vi "Configure.vi"(8 "error in (no error)":errorcluster, 11 "navX - SERIAL in":refnum<class "navX - SERIAL.lvclass">) -> (0 "error out":errorcluster, 3 "navX - SERIAL out":refnum<class "navX - SERIAL.lvclass">)   [LabVIEW 2015, in "navX Library v3.lvlib" / "navX - SERIAL.lvclass"]
uses:
  navX - SERIAL.lvclass
  ProtocolID.ctl
  _NI WPI Serial USB/WPI_SerialPort_USB.ctl
  navX - SERIAL.lvclass/navX - SERIAL.ctl
  navX - Base/navX - Base.lvclass/navX - Base.ctl
  navX - Base/navX - Base.lvclass
  _NI WPI Serial USB/_NI WPI Serial USB.lvlib
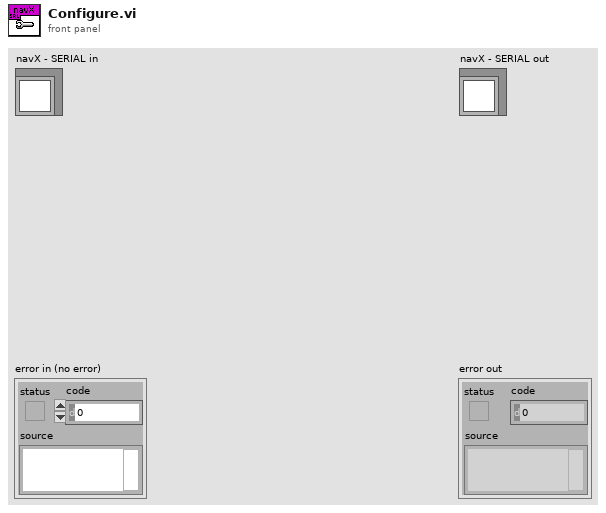
[diagram p1: front panel]
types:
  T1 = typedef "_NI WPI Serial USB.lvlib/WPI_SerialPort_USB.ctl" = enum16{"Onboard RS-232", "MXP TTL", "USB"}
  T2 = typedef "navX Library v3.lvlib/navX - SERIAL.lvclass/ProtocolID.ctl" = string[]
  T3 = typedef "navX Library v3.lvlib/navX - SERIAL.lvclass/Protocol.ctl" = enum16{"YRPH", "Quaterinons", "Gyro/Raw", "AHRS", "AHRSAndPositioning"}
  T4 = typedef "WPI_SerialPortRef.ctl" = cluster{"DevStatus":errorcluster, "Serial Port Name":refnum<visa-resource-name>}
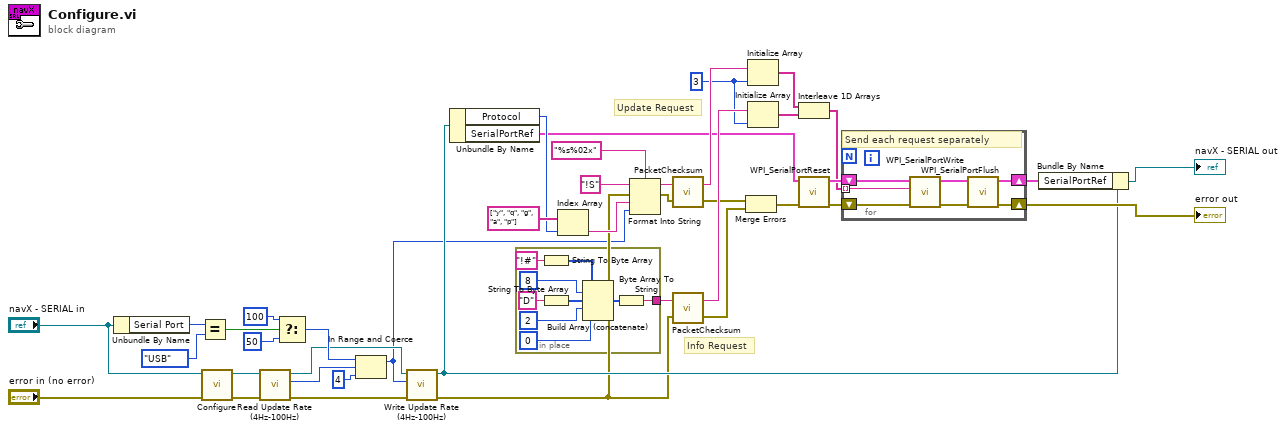
[diagram p0: block diagram]
diagram:
  w23 = 3 ("dimension size")
  # "Info Request"
  # "Update Request"
  n1 = Unbundle By Name("navX - SERIAL in") -> ("Serial Port"=w38:T1)
  n2 = Equal?(x=w38, y=WPI_SerialPort_USB."USB") -> (x = y?=w36:bool)
  n3 = call-parent "Configure.vi"("error in (no error)"="error in (no error)", "navX - Base in"="navX - SERIAL in") -> ("error out"=w6:errorcluster, "navX - Base out"=w7:refnum<class "navX - SERIAL.lvclass">)  [unwired: 8 in]
  n4 = call "Read Update Rate (4Hz-100Hz).vi"("error in (no error)"=w6, "navX - Base in"=w7) -> ("error out"=w4:errorcluster, "Update Rate (4Hz-100Hz)"=w8:u8, "navX - Base out"=w5:refnum<class "navX - SERIAL.lvclass">)  [unwired: 7 in]
  n5 = Select(t=u8 100, s=w36, f=u8 50) -> (s? t:f=w9:u8)
  n6 = In Range and Coerce(upper limit=w9, x=w8, lower limit=u8 4) -> (coerced(x)=w1:u8)  [unwired: 1 out]
  n7 = call "Write Update Rate (4Hz-100Hz).vi"("error in (no error)"=w4, "Update Rate (4Hz-100Hz)"=w1, "navX - Base in"=w5) -> ("error out"=w2:errorcluster, "navX - Base out"=w3:refnum<class "navX - SERIAL.lvclass">)  [unwired: 7 in]
  n8 = Unbundle By Name(w3) -> ("Protocol"=w32:T3, "SerialPortRef"=w17:T4)
  n9 = in-place {
    in-place-border: [w41] -> w25
    n10 = String To Byte Array(string="!#" ("initial string")) -> (unsigned byte array=w47:u8[])
    n11 = String To Byte Array(string="D" ("initial string")) -> (unsigned byte array=w45:u8[])
    n12 = Build Array (concatenate)(w47, 8, w45, 2, 0) -> (w42:i32[])
    n13 = Byte Array To String(unsigned byte array=w42) -> (string=w41:string)
  }
  n14 = Index Array(array=T2 ["y", "q", "g", "a", "p"] ("Protocol IDs"), index=w32) -> (element=w29:string)
  n15 = Format Into String(format string="%s%02x", initial string="!S", error in=w2, w29, w1) -> (resulting string=w28:string, error out=w27:errorcluster)
  n16 = call "PacketChecksum.vi"("error in (no error)"=w27, "Packet"=w28) -> ("error out"=w16:errorcluster, "Terminated Packet"=w26:string)
  n17 = call "PacketChecksum.vi"("error in (no error)"=w2, "Packet"=w25) -> ("error out"=w15:errorcluster, "Terminated Packet"=w24:string)
  n18 = Merge Errors(w16, w15) -> (w14:errorcluster)
  n19 = Initialize Array(w26, w23) -> (w22:string[])
  n20 = Initialize Array(w24, w23) -> (w21:string[])
  n21 = Interleave 1D Arrays(w22, w21) -> (w18:string[])
  n22 = call <vilib>:"WPI_SerialPortReset.vi"("error in (no error)"=w14, "SerialPortRef"=w17) -> ("error out"=w19:errorcluster, "SerialPortRef"=w20:T4)  [unwired: 8 in]
  n23 = for {
    tunnel: w18 -> [w52] mode=indexing
    shift-right: [w50] -> w11
    shift-left: w19 -> [w53]
    shift-right: [w51] -> w12
    shift-left: w20 -> [w54]
    # "Send each request separately"
    n24 = call <vilib>:"WPI_SerialPortWrite.vi"("error in (no error)"=w53, "Buffer"=w52, "SerialPortRef"=w54) -> ("error out"=w55:errorcluster, "SerialPortRef"=w56:T4)  [unwired: 6 in, 1 out]
    n25 = call <vilib>:"WPI_SerialPortFlush.vi"("error in (no error)"=w55, "SerialPortRef"=w56) -> ("error out"=w50:errorcluster, "SerialPortRef"=w51:T4)  [unwired: 8 in]
  }
  "error out" <- w11
  n26 = Bundle By Name(cluster=w3, "SerialPortRef"=w12) -> (→"navX - SERIAL out":refnum<class "navX - SERIAL.lvclass">)
